vi "BRig_RT__Case_Exp__State_initTrial__LC_Select__v4.vi"(6 "input_arrTrig":bool[](array[boolean]), 8 "input_dataTrial":u16[][](array[numeric]), 9 "input_dataExp":u16[](array[numeric]), 10 "input_dataLC":u16[](array[numeric]), 11 "input_dataCurrent":u16[](array[numeric])) -> (0 "output_dataTrial":u16[][](array[numeric]), 3 "output_dataCurrent":u16[](array[numeric]), 4 "output_arrTrig":bool[](array[boolean]))   [LabVIEW 2014]
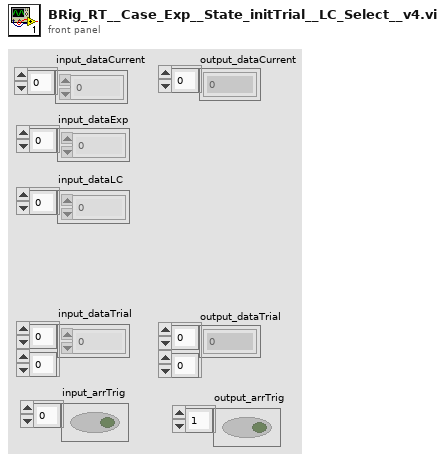
[diagram p1: front panel]
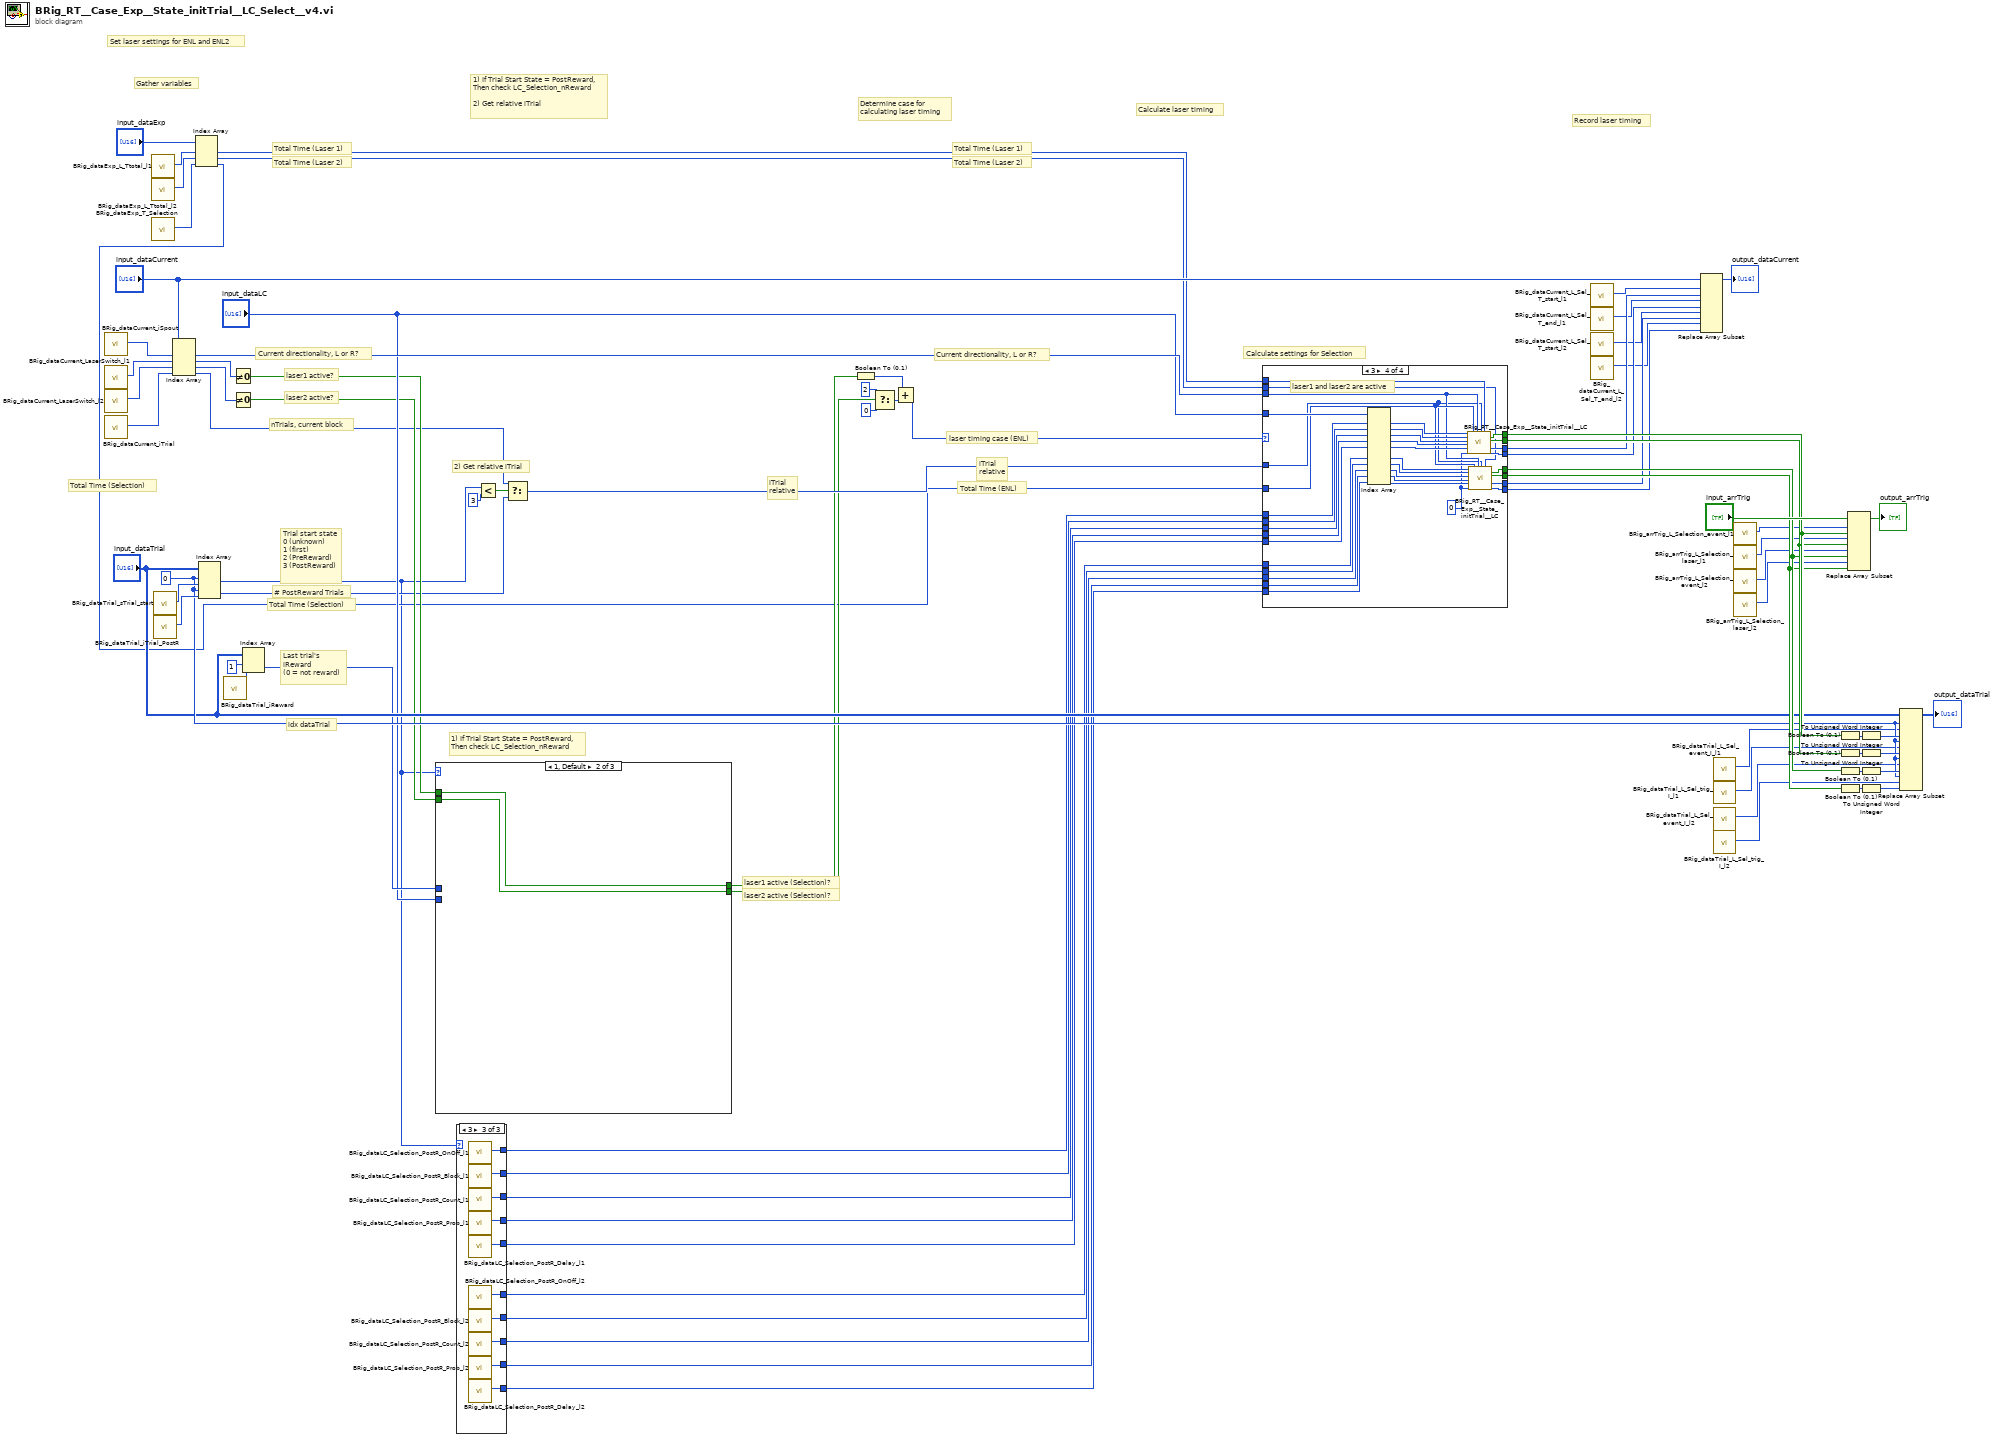
[diagram p0: block diagram]
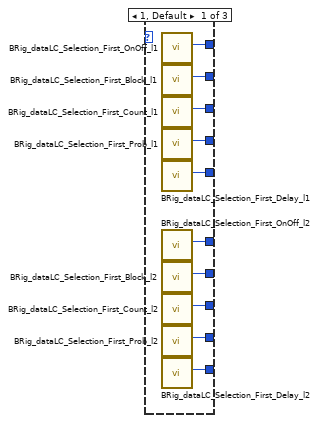
[diagram p2: hidden frame]
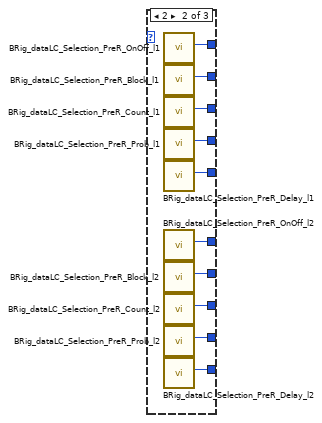
[diagram p3: hidden frame]
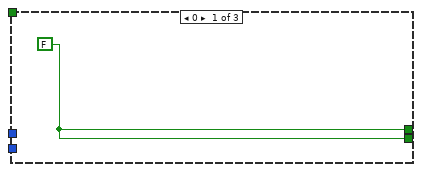
[diagram p4: hidden frame]
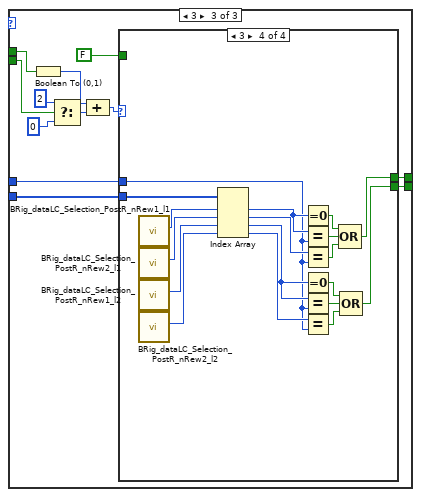
[diagram p5: hidden frame]
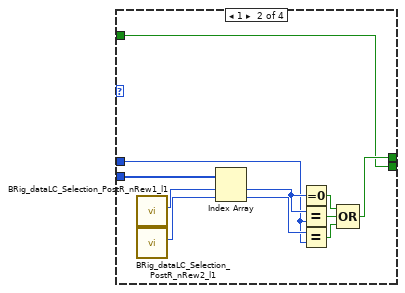
[diagram p7: hidden frame]
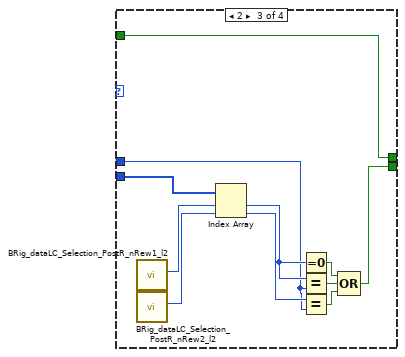
[diagram p8: hidden frame]
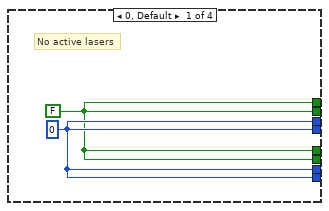
[diagram p9: hidden frame]
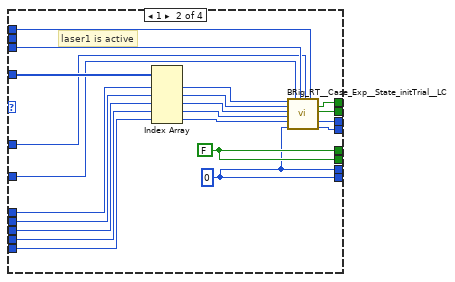
[diagram p10: hidden frame]
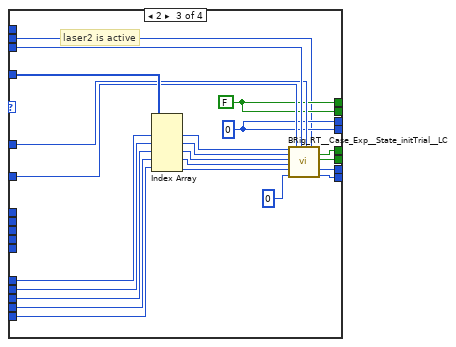
[diagram p11: hidden frame]
diagram:
  w44 = 0
  # "Total Time (Selection)"
  # "Record laser timing"
  # "Calculate laser timing"
  # "Total Time (ENL)"
  # "iTrial\nrelative"
  # "Total Time (Laser 2)"
  # "Total Time (Laser 1)"
  # "Current directionality, L or R?"
  # "Determine case for\ncalculating laser timing"
  # "2) Get relative iTrial"
  # "1) If Trial Start State = PostReward,\nThen check LC_Selection_nReward"
  # "laser2 active (Selection)?"
  # "laser1 active (Selection)?"
  # "1) If Trial Start State = PostReward,\nThen check LC_Selection_nReward\n\n2) Get relative iTrial"
  # "Gather variables"
  # "Last trial's\niReward\n(0 = not reward)"
  # "nTrials, current block"
  # "idx dataTrial"
  # "Total Time (Selection)"
  # "# PostReward Trials"
  # "Current directionality, L or R?"
  # "Total Time (Laser 2)"
  # "Total Time (Laser 1)"
  # "Calculate settings for Selection"
  # "Set laser settings for ENL and ENL2"
  # "iTrial\nrelative"
  # "laser timing case (ENL)"
  # "Trial start state\n0 (unknown)\n1 (first)\n2 (PreReward)\n3 (PostReward)"
  # "laser2 active?"
  # "laser1 active?"
  n1 = call "BRig_dataCurrent_iSpout.vi"() -> ("output_iSpout"=w71:i32)  [unwired: 11 in]
  n2 = call "BRig_dataCurrent_LaserSwitch_l1.vi"() -> ("output_LaserSwitch_l1"=w80:i32)  [unwired: 11 in]
  n3 = call "BRig_dataCurrent_LaserSwitch_l2.vi"() -> ("output_LaserSwitch_l2"=w79:i32)  [unwired: 11 in]
  n4 = call "BRig_dataCurrent_iTrial.vi"() -> ("output_iTrial"=w45:i32)  [unwired: 11 in]
  n5 = call "BRig_dataExp_L_Ttotal_l1.vi"() -> ("output_L_Ttotal_l1"=w48:i32)  [unwired: 11 in]
  n6 = call "BRig_dataExp_L_Ttotal_l2.vi"() -> ("output_L_Ttotal_l2"=w49:i32)  [unwired: 11 in]
  n7 = call "BRig_dataExp_T_Selection.vi"() -> ("output_T_Selection"=w25:i32)  [unwired: 11 in]
  n8 = call "BRig_dataTrial_sTrial_start.vi"() -> ("output_sTrial_start"=w76:i32)  [unwired: 11 in]
  n9 = call "BRig_dataTrial_iTrial_PostR.vi"() -> ("output_iTrial_PostR"=w46:i32)  [unwired: 11 in]
  n10 = Index Array(array="input_dataCurrent", index #1=w71, index #2=w80, index #3=w79, index #4=w45) -> (element #1=w41:u16, element #2=w78:u16, element #3=w77:u16, element #4=w31:u16)
  n11 = Index Array(array="input_dataExp", index #1=w48, index #2=w49, index #3=w25) -> (element #1=w43:u16, element #2=w42:u16, element #3=w24:u16)
  n12 = Index Array(array="input_dataTrial", index (row) #1=w44, index (col) #1=w76, index (row) #2=w44, index (col) #2=w46) -> (element #1=w23:u16, element #2=w30:u16)
  n13 = call "BRig_dataTrial_iReward.vi"() -> ("output_iReward"=w39:i32)  [unwired: 11 in]
  n14 = Not Equal To 0?(x=w78) -> (x != 0?=w34:bool)
  n15 = Not Equal To 0?(x=w77) -> (x != 0?=w35:bool)
  n16 = Index Array(array="input_dataTrial", index (row)=1 ("disabled index (row)"), index (col)=w39) -> (element=w37:u16)
  n17 = case shown="1, Default" w23 {
    tunnel: w37 -> [_ _ w89]
    tunnel: "input_dataLC" -> [_ _ w90]
    tunnel: w35 -> [_ w82 w84]
    tunnel: w34 -> [_ w83 w85]
    tunnel: [w81 w83 w88] -> w28
    tunnel: [w81 w82 w87] -> w27
    frame 0 {
      w81 = FALSE
    }
    frame 1, Default {
    }
    frame 3 {
      n18 = Boolean To (0,1)(Boolean=w85) -> (0, 1=w92:i16)
      n19 = Select(t=i16 2, s=w84, f=i16 0) -> (s? t:f=w93:i16)
      n20 = Compound Arithmetic op=ADD(w92, w93) -> (w91:i16)
      n21 = case shown="3" w91 {
        tunnel: w90 -> [_ w102 w113 w126]
        tunnel: w89 -> [_ w101 w112 w125]
        tunnel: [w96 w100 w110 w124] -> w88
        tunnel: [w96 w99 w111 w123] -> w87
        tunnel: FALSE -> [w96 w99 w110 _]
        frame 0, Default {
        }
        frame 1 {
          n22 = call "BRig_dataLC_Selection_PostR_nRew1_l1.vi"() -> ("output_Selection_PostR_nRew1_l1"=w97:i32)  [unwired: 11 in]
          n23 = call "BRig_dataLC_Selection_PostR_nRew2_l1.vi"() -> ("output_Selection_PostR_nRew2_l1"=w98:i32)  [unwired: 11 in]
          n24 = Index Array(array=w102, index #1=w97, index #2=w98) -> (element #1=w104:u16, element #2=w103:u16)
          n25 = Equal To 0?(x=w104) -> (x = 0?=w105:bool)
          n26 = Equal?(x=w104, y=w101) -> (x = y?=w106:bool)
          n27 = Equal?(x=w103, y=w101) -> (x = y?=w107:bool)
          n28 = Compound Arithmetic op=OR(w105, w106, w107) -> (w100:bool)
        }
        frame 2 {
          n29 = call "BRig_dataLC_Selection_PostR_nRew1_l2.vi"() -> ("output_Selection_PostR_nRew1_l2"=w108:i32)  [unwired: 11 in]
          n30 = call "BRig_dataLC_Selection_PostR_nRew2_l2.vi"() -> ("output_Selection_PostR_nRew2_l2"=w109:i32)  [unwired: 11 in]
          n31 = Index Array(array=w113, index #1=w108, index #2=w109) -> (element #1=w114:u16, element #2=w115:u16)
          n32 = Equal To 0?(x=w114) -> (x = 0?=w117:bool)
          n33 = Equal?(x=w114, y=w112) -> (x = y?=w116:bool)
          n34 = Equal?(x=w115, y=w112) -> (x = y?=w118:bool)
          n35 = Compound Arithmetic op=OR(w117, w116, w118) -> (w111:bool)
        }
        frame 3 {
          n36 = call "BRig_dataLC_Selection_PostR_nRew1_l1.vi"() -> ("output_Selection_PostR_nRew1_l1"=w119:i32)  [unwired: 11 in]
          n37 = call "BRig_dataLC_Selection_PostR_nRew2_l1.vi"() -> ("output_Selection_PostR_nRew2_l1"=w120:i32)  [unwired: 11 in]
          n38 = call "BRig_dataLC_Selection_PostR_nRew1_l2.vi"() -> ("output_Selection_PostR_nRew1_l2"=w121:i32)  [unwired: 11 in]
          n39 = call "BRig_dataLC_Selection_PostR_nRew2_l2.vi"() -> ("output_Selection_PostR_nRew2_l2"=w122:i32)  [unwired: 11 in]
          n40 = Index Array(array=w126, index #1=w119, index #2=w120, index #3=w121, index #4=w122) -> (element #1=w130:u16, element #2=w129:u16, element #3=w127:u16, element #4=w128:u16)
          n41 = Equal To 0?(x=w130) -> (x = 0?=w131:bool)
          n42 = Equal?(x=w130, y=w125) -> (x = y?=w132:bool)
          n43 = Equal?(x=w129, y=w125) -> (x = y?=w133:bool)
          n44 = Equal To 0?(x=w127) -> (x = 0?=w135:bool)
          n45 = Equal?(x=w127, y=w125) -> (x = y?=w134:bool)
          n46 = Equal?(x=w128, y=w125) -> (x = y?=w136:bool)
          n47 = Compound Arithmetic op=OR(w131, w132, w133) -> (w124:bool)
          n48 = Compound Arithmetic op=OR(w135, w134, w136) -> (w123:bool)
        }
      }
    }
  }
  n49 = case shown="3" w23 {
    tunnel: [w146 w156 w166] -> w22
    tunnel: [w139 w154 w164] -> w21
    tunnel: [w140 w153 w163] -> w20
    tunnel: [w141 w152 w162] -> w19
    tunnel: [w142 w151 w161] -> w18
    tunnel: [w145 w155 w165] -> w17
    tunnel: [w143 w150 w160] -> w16
    tunnel: [w144 w149 w159] -> w15
    tunnel: [w137 w148 w158] -> w14
    tunnel: [w138 w147 w157] -> w13
    frame 1, Default {
      n50 = call "BRig_dataLC_Selection_First_OnOff_l1.vi"() -> ("output_Selection_First_OnOff"=w146:i32)  [unwired: 11 in]
      n51 = call "BRig_dataLC_Selection_First_Block_l1.vi"() -> ("output_Selection_First_Block"=w139:i32)  [unwired: 11 in]
      n52 = call "BRig_dataLC_Selection_First_Count_l1.vi"() -> ("output_Selection_First_Count"=w140:i32)  [unwired: 11 in]
      n53 = call "BRig_dataLC_Selection_First_Prob_l1.vi"() -> ("output_Selection_First_Prob"=w141:i32)  [unwired: 11 in]
      n54 = call "BRig_dataLC_Selection_First_Delay_l1.vi"() -> ("output_Selection_First_Delay"=w142:i32)  [unwired: 11 in]
      n55 = call "BRig_dataLC_Selection_First_OnOff_l2.vi"() -> ("output_Selection_First_OnOff_l2"=w145:i32)  [unwired: 11 in]
      n56 = call "BRig_dataLC_Selection_First_Block_l2.vi"() -> ("output_Selection_First_Block_l2"=w143:i32)  [unwired: 11 in]
      n57 = call "BRig_dataLC_Selection_First_Count_l2.vi"() -> ("output_Selection_First_Count_l2"=w144:i32)  [unwired: 11 in]
      n58 = call "BRig_dataLC_Selection_First_Prob_l2.vi"() -> ("output_Selection_First_Prob_l2"=w137:i32)  [unwired: 11 in]
      n59 = call "BRig_dataLC_Selection_First_Delay_l2.vi"() -> ("output_Selection_First_Delay_l2"=w138:i32)  [unwired: 11 in]
    }
    frame 2 {
      n60 = call "BRig_dataLC_Selection_PreR_OnOff_l1.vi"() -> ("output_Selection_PreR_OnOff"=w156:i32)  [unwired: 11 in]
      n61 = call "BRig_dataLC_Selection_PreR_Block_l1.vi"() -> ("output_Selection_PreR_Block"=w154:i32)  [unwired: 11 in]
      n62 = call "BRig_dataLC_Selection_PreR_Count_l1.vi"() -> ("output_Selection_PreR_Count"=w153:i32)  [unwired: 11 in]
      n63 = call "BRig_dataLC_Selection_PreR_Prob_l1.vi"() -> ("output_Selection_PreR_Prob"=w152:i32)  [unwired: 11 in]
      n64 = call "BRig_dataLC_Selection_PreR_Delay_l1.vi"() -> ("output_Selection_PreR_Delay"=w151:i32)  [unwired: 11 in]
      n65 = call "BRig_dataLC_Selection_PreR_OnOff_l2.vi"() -> ("output_Selection_PreR_OnOff_l2"=w155:i32)  [unwired: 11 in]
      n66 = call "BRig_dataLC_Selection_PreR_Block_l2.vi"() -> ("output_Selection_PreR_Block_l2"=w150:i32)  [unwired: 11 in]
      n67 = call "BRig_dataLC_Selection_PreR_Count_l2.vi"() -> ("output_Selection_PreR_Count_l2"=w149:i32)  [unwired: 11 in]
      n68 = call "BRig_dataLC_Selection_PreR_Prob_l2.vi"() -> ("output_Selection_PreR_Prob_l2"=w148:i32)  [unwired: 11 in]
      n69 = call "BRig_dataLC_Selection_PreR_Delay_l2.vi"() -> ("output_Selection_PreR_Delay_l2"=w147:i32)  [unwired: 11 in]
    }
    frame 3 {
      n70 = call "BRig_dataLC_Selection_PostR_OnOff_l1.vi"() -> ("output_Selection_PostR_OnOff"=w166:i32)  [unwired: 11 in]
      n71 = call "BRig_dataLC_Selection_PostR_Block_l1.vi"() -> ("output_Selection_PostR_Block"=w164:i32)  [unwired: 11 in]
      n72 = call "BRig_dataLC_Selection_PostR_Count_l1.vi"() -> ("output_Selection_PostR_Count"=w163:i32)  [unwired: 11 in]
      n73 = call "BRig_dataLC_Selection_PostR_Prob_l1.vi"() -> ("output_Selection_PostR_Prob"=w162:i32)  [unwired: 11 in]
      n74 = call "BRig_dataLC_Selection_PostR_Delay_l1.vi"() -> ("output_Selection_PostR_Delay"=w161:i32)  [unwired: 11 in]
      n75 = call "BRig_dataLC_Selection_PostR_OnOff_l2.vi"() -> ("output_Selection_PostR_OnOff_l2"=w165:i32)  [unwired: 11 in]
      n76 = call "BRig_dataLC_Selection_PostR_Block_l2.vi"() -> ("output_Selection_PostR_Block_l2"=w160:i32)  [unwired: 11 in]
      n77 = call "BRig_dataLC_Selection_PostR_Count_l2.vi"() -> ("output_Selection_PostR_Count_l2"=w159:i32)  [unwired: 11 in]
      n78 = call "BRig_dataLC_Selection_PostR_Prob_l2.vi"() -> ("output_Selection_PostR_Prob_l2"=w158:i32)  [unwired: 11 in]
      n79 = call "BRig_dataLC_Selection_PostR_Delay_l2.vi"() -> ("output_Selection_PostR_Delay_l2"=w157:i32)  [unwired: 11 in]
    }
  }
  n80 = Less?(x=w23, y=u16 3) -> (x < y?=w32:bool)
  n81 = Select(t=w31, s=w32, f=w30) -> (s? t:f=w29:u16)
  n82 = Boolean To (0,1)(Boolean=w28) -> (0, 1=w73:i16)
  n83 = Select(t=i16 2, s=w27, f=i16 0) -> (s? t:f=w74:i16)
  n84 = Add(x=w73, y=w74) -> (x+y=w26:i16)
  n85 = case shown="3" w26 {
    tunnel: "input_dataLC" -> [_ w189 w211 w246]
    tunnel: w41 -> [_ w182 w204 w234]
    tunnel: w24 -> [_ w183 w205 w235]
    tunnel: w29 -> [_ w181 w203 w233]
    tunnel: [w167 w180 w193 w232] -> w64
    tunnel: [w167 w179 w193 w231] -> w61
    tunnel: [w168 w178 w192 w230] -> w53
    tunnel: [w168 w177 w192 w229] -> w52
    tunnel: [w167 w171 w202 w228] -> w57
    tunnel: [w168 w169 w201 w227] -> w51
    tunnel: [w167 w171 w200 w226] -> w59
    tunnel: [w168 w169 w199 w225] -> w50
    tunnel: w22 -> [_ w176 _ w224]
    tunnel: w21 -> [_ w175 _ w223]
    tunnel: w20 -> [_ w174 _ w222]
    tunnel: w19 -> [_ w173 _ w221]
    tunnel: w18 -> [_ w172 _ w220]
    tunnel: w17 -> [_ _ w198 w219]
    tunnel: w16 -> [_ _ w197 w218]
    tunnel: w15 -> [_ _ w196 w217]
    tunnel: w14 -> [_ _ w195 w216]
    tunnel: w13 -> [_ _ w194 w215]
    tunnel: w43 -> [_ w170 _ w214]
    tunnel: w42 -> [_ _ w191 w213]
    frame 0, Default {
      w168 = u16 0
      w167 = FALSE
      # "No active lasers"
    }
    frame 1 {
      w169 = u16 0
      w171 = FALSE
      # "laser1 is active"
      n86 = Index Array(array=w189, index #1=w176, index #2=w175, index #3=w174, index #4=w173, index #5=w172) -> (element #1=w188:u16, element #2=w187:u16, element #3=w186:u16, element #4=w185:u16, element #5=w184:u16)
      n87 = call "BRig_RT__Case_Exp__State_initTrial__LC.vi"("input_L_OnOff"=w188, "input_L_Block"=w187, "input_L_Count"=w186, "input_L_Prob"=w185, "input_L_Tdelay"=w184, "input_L_delayOpt"=w169, "input_T_state"=w183, "input_iSpout"=w182, "input_iTrial_relative"=w181, "input_L_T"=w170) -> ("output_LC_Event"=w180:bool, "output_LC_Laser"=w179:bool, "output_L_Tstart"=w178:u16, "output_L_Tend"=w177:u16)  [unwired: 6 in]
    }
    frame 2 {
      w192 = u16 0
      w193 = FALSE
      # "laser2 is active"
      n88 = Index Array(array=w211, index #1=w198, index #2=w197, index #3=w196, index #4=w195, index #5=w194) -> (element #1=w206:u16, element #2=w207:u16, element #3=w208:u16, element #4=w209:u16, element #5=w210:u16)
      n89 = call "BRig_RT__Case_Exp__State_initTrial__LC.vi"("input_L_OnOff"=w206, "input_L_Block"=w207, "input_L_Count"=w208, "input_L_Prob"=w209, "input_L_Tdelay"=w210, "input_L_delayOpt"=u16 0, "input_T_state"=w205, "input_iSpout"=w204, "input_iTrial_relative"=w203, "input_L_T"=w191) -> ("output_LC_Event"=w200:bool, "output_LC_Laser"=w202:bool, "output_L_Tstart"=w201:u16, "output_L_Tend"=w199:u16)  [unwired: 6 in]
    }
    frame 3 {
      w212 = u16 0 ("input_L_delayOpt")
      # "laser1 and laser2 are active"
      n90 = Index Array(array=w246, index #1=w224, index #2=w223, index #3=w222, index #4=w221, index #5=w220, index #7=w219, index #8=w218, index #9=w217, index #10=w216, index #11=w215) -> (element #1=w245:u16, element #2=w244:u16, element #3=w243:u16, element #4=w242:u16, element #5=w241:u16, element #7=w236:u16, element #8=w237:u16, element #9=w238:u16, element #10=w239:u16, element #11=w240:u16)  [unwired: 1 in, 1 out]
      n91 = call "BRig_RT__Case_Exp__State_initTrial__LC.vi"("input_L_OnOff"=w245, "input_L_Block"=w244, "input_L_Count"=w243, "input_L_Prob"=w242, "input_L_Tdelay"=w241, "input_L_delayOpt"=w212, "input_T_state"=w235, "input_iSpout"=w234, "input_iTrial_relative"=w233, "input_L_T"=w214) -> ("output_LC_Event"=w232:bool, "output_LC_Laser"=w231:bool, "output_L_Tstart"=w230:u16, "output_L_Tend"=w229:u16)  [unwired: 6 in]
      n92 = call "BRig_RT__Case_Exp__State_initTrial__LC.vi"("input_L_OnOff"=w236, "input_L_Block"=w237, "input_L_Count"=w238, "input_L_Prob"=w239, "input_L_Tdelay"=w240, "input_L_delayOpt"=w212, "input_T_state"=w235, "input_iSpout"=w234, "input_iTrial_relative"=w233, "input_L_T"=w213) -> ("output_LC_Event"=w226:bool, "output_LC_Laser"=w228:bool, "output_L_Tstart"=w227:u16, "output_L_Tend"=w225:u16)  [unwired: 6 in]
    }
  }
  n93 = call "BRig_dataCurrent_L_Sel_T_start_l1.vi"() -> ("output_L_Sel_T_start_l1"=w9:i32)  [unwired: 11 in]
  n94 = call "BRig_dataCurrent_L_Sel_T_end_l1.vi"() -> ("output_L_Sel_T_end_l1"=w10:i32)  [unwired: 11 in]
  n95 = call "BRig_dataCurrent_L_Sel_T_start_l2.vi"() -> ("output_L_Sel_T_start_l2"=w11:i32)  [unwired: 11 in]
  n96 = call "BRig_dataCurrent_L_Sel_T_end_l2.vi"() -> ("output_L_Sel_T_end_l2"=w12:i32)  [unwired: 11 in]
  n97 = Replace Array Subset(array="input_dataCurrent", new element #1=w53, index #1=w9, new element #2=w52, index #2=w10, new element #3=w51, index #3=w11, new element #4=w50, index #4=w12) -> (→"output_dataCurrent":u16[])
  n98 = call "BRig_dataTrial_L_Sel_event_I_l1.vi"() -> ("output_L_Sel_event_I_l1"=w4:i32)  [unwired: 11 in]
  n99 = call "BRig_dataTrial_L_Sel_trig_I_l1.vi"() -> ("output_L_Sel_trig_I_l1"=w3:i32)  [unwired: 11 in]
  n100 = call "BRig_dataTrial_L_Sel_event_I_l2.vi"() -> ("output_L_Sel_event_I_l2"=w2:i32)  [unwired: 11 in]
  n101 = call "BRig_dataTrial_L_Sel_trig_I_l2.vi"() -> ("output_L_Sel_trig_I_l2"=w1:i32)  [unwired: 11 in]
  n102 = call "BRig_arrTrig_L_Selection_event_l1.vi"() -> ("output_L_Sel_event_l1"=w5:i32)  [unwired: 11 in]
  n103 = call "BRig_arrTrig_L_Selection_laser_l1.vi"() -> ("output_L_Sel_laserTrig_l1"=w6:i32)  [unwired: 11 in]
  n104 = call "BRig_arrTrig_L_Selection_event_l2.vi"() -> ("output_L_Sel_event_l2"=w7:i32)  [unwired: 11 in]
  n105 = call "BRig_arrTrig_L_Selection_laser_l2.vi"() -> ("output_L_Sel_laserTrig_l2"=w8:i32)  [unwired: 11 in]
  n106 = Boolean To (0,1)(Boolean=w64) -> (0, 1=w68:i16)
  n107 = Boolean To (0,1)(Boolean=w61) -> (0, 1=w67:i16)
  n108 = Boolean To (0,1)(Boolean=w59) -> (0, 1=w65:i16)
  n109 = Boolean To (0,1)(Boolean=w57) -> (0, 1=w66:i16)
  n110 = Replace Array Subset(array="input_arrTrig", new element #1=w64, index #1=w5, new element #2=w61, index #2=w6, new element #3=w59, index #3=w7, new element #4=w57, index #4=w8) -> (→"output_arrTrig":bool[])
  n111 = To Unsigned Word Integer(number=w68) -> (unsigned 16bit integer=w63:u16)
  n112 = To Unsigned Word Integer(number=w67) -> (unsigned 16bit integer=w62:u16)
  n113 = To Unsigned Word Integer(number=w65) -> (unsigned 16bit integer=w60:u16)
  n114 = To Unsigned Word Integer(number=w66) -> (unsigned 16bit integer=w58:u16)
  n115 = Replace Array Subset(array="input_dataTrial", new element #1=w63, index (row) #1=w44, index (col) #1=w4, new element #2=w62, index (row) #2=w44, index (col) #2=w3, new element #3=w60, index (row) #3=w44, index (col) #3=w2, new element #4=w58, index (row) #4=w44, index (col) #4=w1) -> (→"output_dataTrial":u16[][])
